vi "parse_simulator_version.vi"(4 "error in":errorcluster, 7 "Response JSON":string="{\"message\":\"simulator_version: 1.11.0, api_version: 4.0\",\"reference\":1111,\"success\":true,\"type\":\"GetVersion\"}") -> (0 "error out":errorcluster, 2 "Simulator version":string, 3 "API version":string)   [LabVIEW 2025]
doc: "Obtain the simulator's current version and the current API version"
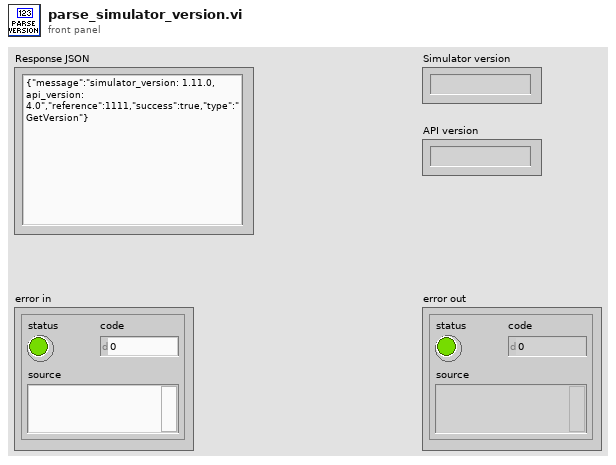
[diagram p1: front panel]
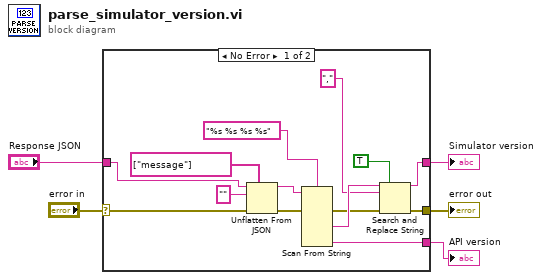
[diagram p0: block diagram]
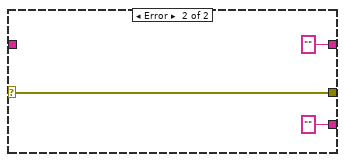
[diagram p2: hidden frame]
diagram:
  n1 = case shown="No Error" "error in" {
    selector: "error in" -> [w17 w22]
    tunnel: [w10 w22] -> w5
    tunnel: [w7 "" ("after match")] -> w3
    tunnel: [w6 "" ("after match")] -> w2
    tunnel: "Response JSON" -> [w16 _]
    frame No Error {
      n2 = Unflatten From JSON(path=string[] ["message"], JSON string=w16, type and defaults="", error in (no error)=w17) -> (value=w14:string, error out=w13:errorcluster)  [unwired: 3 in]
      n3 = Scan From String(format string="%s %s %s %s", input string=w14, error in=w13) -> (error out=w11:errorcluster, output 2=w12:string, output 4=w6:string)  [unwired: 7 in, 2 out]
      n4 = Search and Replace String(replace all?=TRUE ("replace all? (F)"), input string=w12, search string=",", error in=w11) -> (result string=w7:string, error out=w10:errorcluster)  [unwired: 4 in, 2 out]
    }
    frame Error {
    }
  }
  "error out" <- w5
  "Simulator version" <- w3
  "API version" <- w2
